vi "begin direct write.vi"(7 "id":u32, 8 "error in":errorcluster, 10 "data":string, 11 "connection in":refnum<class "connection.lvclass">) -> (0 "error out":errorcluster)   [LabVIEW 2016, in "connection.lvclass"]
uses:
  connection.lvclass
  connection.lvclass/connection.ctl
  dllwrapper/library path.vi
  <vilib>/Utility/error.llb/Error Cluster From Error Code.vi
  dllwrapper/async tls dl.lvlib
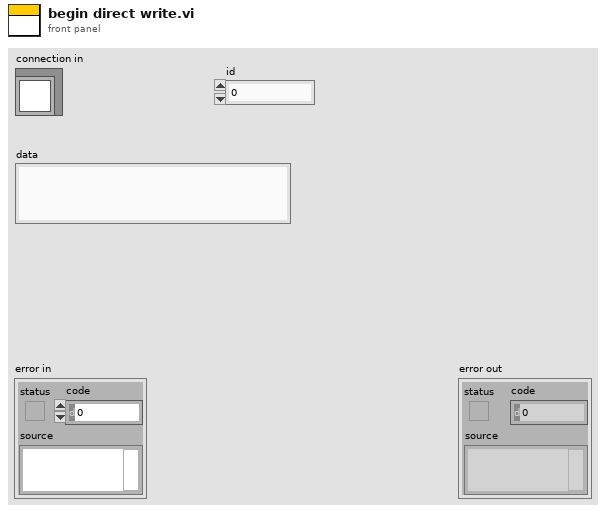
[diagram p1: front panel]
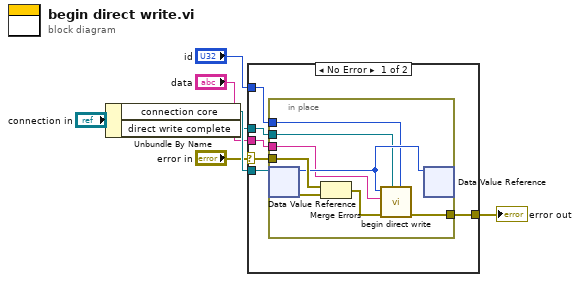
[diagram p0: block diagram]
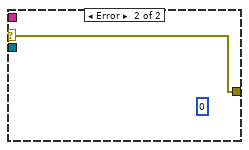
[diagram p2: hidden frame]
diagram:
  n1 = Unbundle By Name("connection in") -> ("connection core"=w6:refnum<data-value>, "direct write complete"=w3:refnum<user-event>)
  n2 = case shown="No Error" "error in" {
    selector: "error in" -> [w12 w22]
    tunnel: w6 -> [w13 _]
    tunnel: [w11 w22] -> w4
    tunnel: w3 -> [w10 _]
    tunnel: "id" -> [w9 _]
    tunnel: "data" -> [w8 _]
    frame No Error {
      n3 = in-place {
        in-place-border: w12 -> [w21]
        in-place-border: [w18] -> w11
        in-place-border: w10 -> [w16]
        in-place-border: w9 -> [w15]
        in-place-border: w8 -> [w14]
        n4 = in-place-dvr #1(w13) -> (w17:u64, w20:errorcluster)
        n5 = Merge Errors(w21, w20) -> (w19:errorcluster)
        n6 = call "begin direct write.vi"("requestID"=w15, "event"=w16, "error in"=w19, "data"=w14, "socket"=w17) -> ("error out"=w18:errorcluster)  [unwired: 6 in]
        n7 = in-place-dvr #1(w17) -> ()  [unwired: 2 out]
      }
    }
    frame Error {
      (unwired) u64 0 ("size")
    }
  }
  "error out" <- w4
